vi "all_images_2_text(+cut).vi"() -> ()   [LabVIEW 2015]
uses:
  <vilib>/picture/picture.llb/Draw True-Color Pixmap.vi
panel:
  out "appended path":path
  out "new":u8[][](array[numeric]) format="%x"
  in  "Cate poze ai?":i32
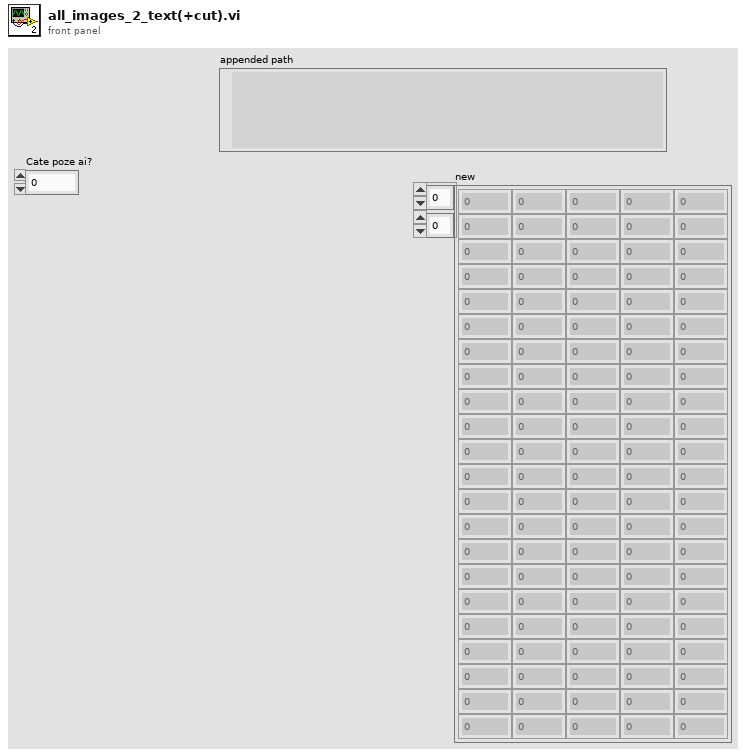
[diagram p1: front panel]
types:
  T1 = typedef "imagedata.ctl" = cluster{"image type":i32, "image depth":i32, "image":u8[], "mask":u8[], "colors":u32[], "Rectangle":cluster{"left":i16, "top":i16, "right":i16, "bottom":i16}}
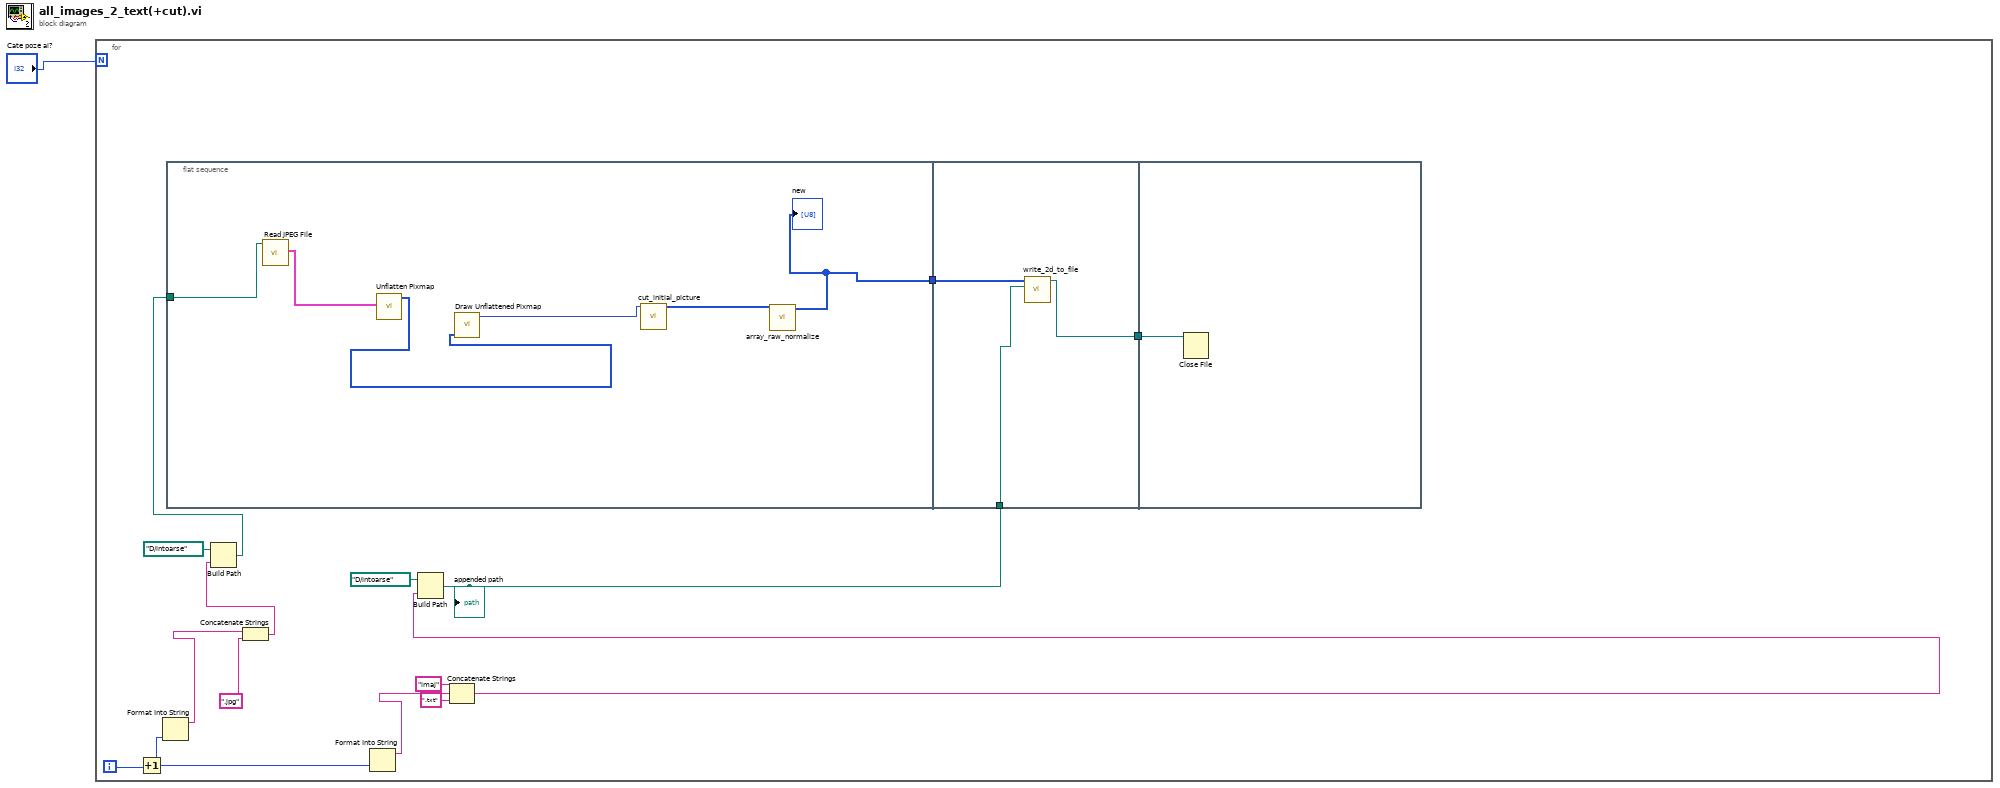
[diagram p0: block diagram]
diagram:
  n1 = for {
    N: "Cate poze ai?" -> [_]
    i -> [w4]
    n2 = Increment(x=w4) -> (x+1=w3:i32)
    n3 = Format Into String(w3) -> (resulting string=w15:string)  [unwired: 3 in, 1 out]
    n4 = flat-sequence {
      tunnel: [w18] -> w8
      tunnel: w6 -> [w21]
      tunnel: w8 -> [w25]
      tunnel: [w24] -> w7
      tunnel: w5 -> [w23]
      tunnel: w7 -> [w26]
      frame #0 {
        n5 = call <vilib>:"Read JPEG File.vi"("path to JPEG file"=w21) -> ("image data"=w20:T1)  [unwired: 8 in, 2 out]
        n6 = call <vilib>:"Unflatten Pixmap.vi"("image data"=w20) -> ("24-bit pixmap"=w17:u32[][])  [unwired: 4 in, 6 out]
        n7 = call-poly <vilib>:"Draw Unflattened Pixmap.vi"("data (RGB format)"=w17) -> ("new picture"=w22:picture)  [unwired: 8 in]
        n8 = call "cut_initial_picture.vi"("picture"=w22) -> ("new"=w19:u32[][])  [unwired: 14 in]
        n9 = call "array_raw_normalize.vi"("array"=w19) -> ("Array"=w18:u8[][])  [unwired: 10 in]
        "new" <- w18
      }
      frame #1 {
        n10 = call "write_2d_to_file.vi"("Path 2"=w23, "Array"=w25) -> ("refnum out"=w24:refnum<file>)  [unwired: 9 in]
      }
      frame #2 {
        n11 = Close File(refnum=w26) -> ()  [unwired: 1 in, 2 out]
      }
    }
    n12 = Concatenate Strings(w15, ".jpg" ("string")) -> (w13:string)
    n13 = Build Path(base path=path "D:/intoarse", name or relative path=w13) -> (appended path=w6:path)
    n14 = Format Into String(w3) -> (resulting string=w11:string)  [unwired: 3 in, 1 out]
    n15 = Concatenate Strings("imaj" ("string"), w11, ".txt" ("string")) -> (w9:string)
    n16 = Build Path(base path=path "D:/intoarse", name or relative path=w9) -> (appended path=w5:path)
    "appended path" <- w5
  }
